vi "LoadPlanckianLocus.vi"(11 "relative path":string) -> (2 "Planckian locus":cluster{"all rows":dbl[], "all rows":dbl[]}, 3 "CCTs":dbl[](array[numeric]))   [LabVIEW 2011]
uses:
  <vilib>/Utility/file.llb/Read From Spreadsheet File (DBL).vi
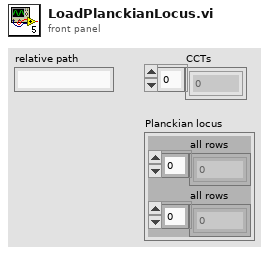
[diagram p1: front panel]
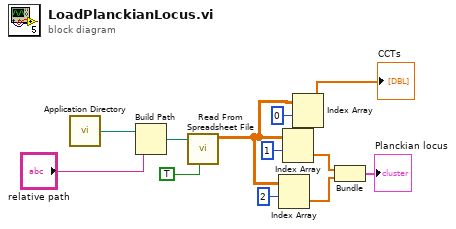
[diagram p0: block diagram]
diagram:
  n1 = call <vilib>:"Application Directory.vi"() -> ("Application Directory"=w1:path)
  n2 = Build Path(base path=w1, name or relative path="relative path") -> (appended path=w2:path)
  n3 = call-poly <vilib>:"Read From Spreadsheet File.vi"("transpose (no:F)"=TRUE, "file path (dialog if empty)"=w2) -> ("all rows"=w11:dbl[][])  [unwired: 5 in, 4 out]
  n4 = Index Array(array=w11, index (row)=2) -> (element=w7:dbl[])  [unwired: 1 in]
  n5 = Index Array(array=w11, index (row)=1) -> (element=w6:dbl[])  [unwired: 1 in]
  n6 = Index Array(array=w11, index (row)=0) -> (element=→"CCTs":dbl[])  [unwired: 1 in]
  n7 = Bundle("all rows"=w6, "all rows"=w7) -> (→"Planckian locus":cluster{"all rows":dbl[], "all rows":dbl[]})  [unwired: 1 in]
